vi "WaitMachine2OFF.vi"(10 "Station":string, 11 "SN":string="7510833") -> (0 "DupResult":string, 1 "Result":string, 2 "NGTag":string, 3 "Left/Right":string)   [LabVIEW 2020]
uses:
  <vilib>/Utility/config.llb/Read Key (String).vi
  <vilib>/Utility/config.llb/NI_LVConfig.lvlib
panel:
  out "Running":bool
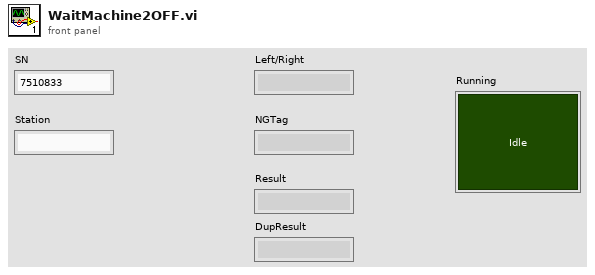
[diagram p1: front panel]
types:
  T1 = typedef "NI_LVConfig.lvlib/Config Data RefNum.ctl" = refnum<k1>
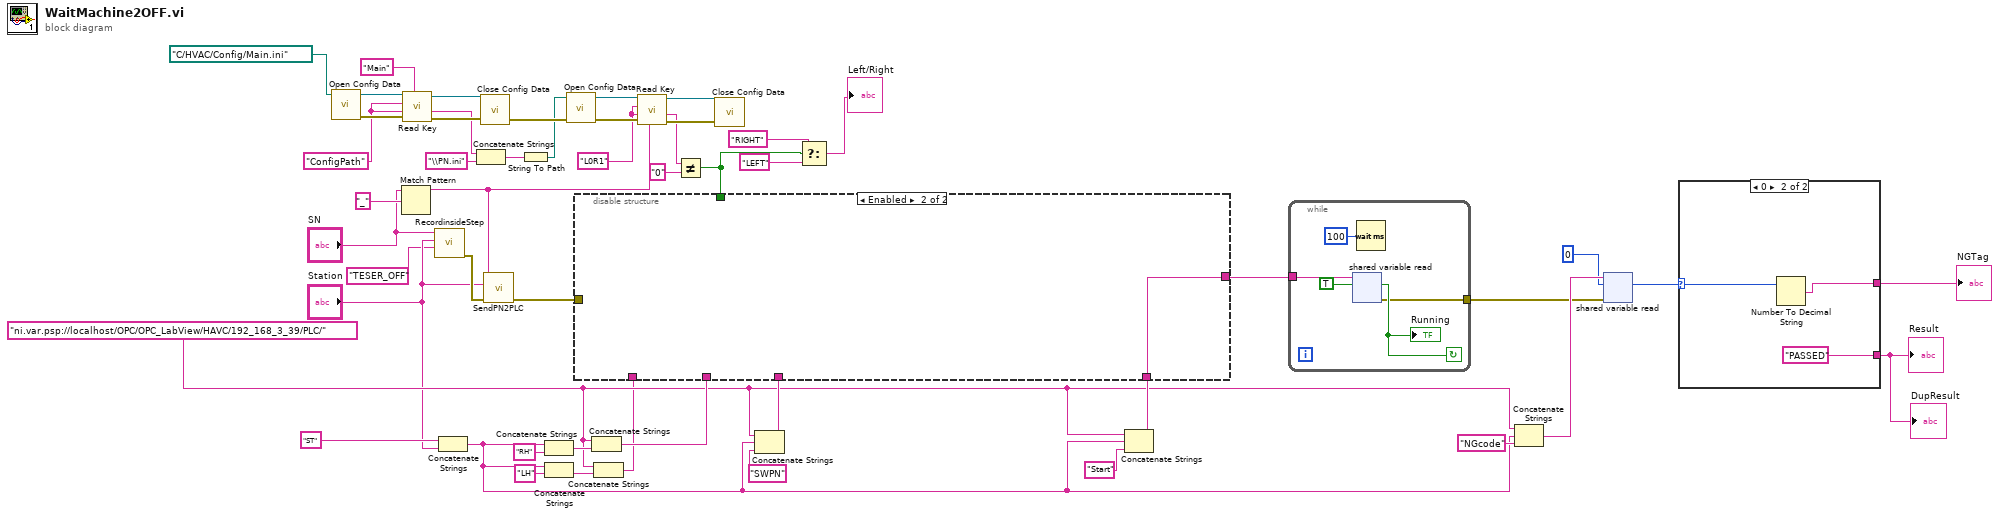
[diagram p0: block diagram]
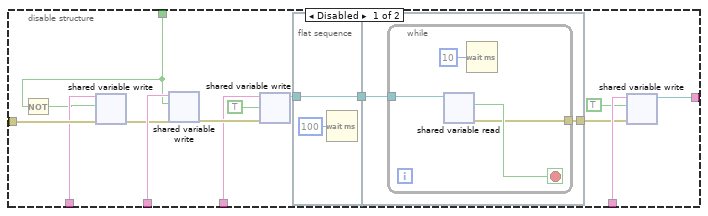
[diagram p2: hidden frame]
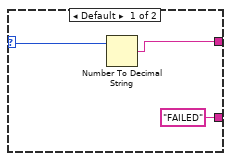
[diagram p3: hidden frame]
diagram:
  w31 = "L0R1"
  w45 = "ConfigPath" ("key")
  w10 = "ni.var.psp://localhost/OPC/OPC_LabView/HAVC/192_168_3_39/PLC/" ("string")
  n1 = call <vilib>:"Open Config Data.vi"("configuration file path"=path "C:/HVAC/Config/Main.ini") -> ("error out"=w50:errorcluster, "refnum"=w49:T1)  [unwired: 8 in, 1 out]
  n2 = Match Pattern(string="SN", regular expression="_") -> (before substring=w6:string)  [unwired: 1 in, 3 out]
  n3 = call-poly <vilib>:"Read Key.vi"("section"="Main", "error in (no error)"=w50, "default value"=w45, "key"=w45, "refnum"=w49) -> ("error out"=w47:errorcluster, "value"=w44:string, "refnum out"=w48:T1)  [unwired: 3 in, 1 out]
  n4 = call "RecordinsideStep.vi"("STEP"="TESER_OFF", "Station"="Station", "SN"="SN") -> ("error out"=w4:errorcluster)  [unwired: 8 in]
  n5 = Concatenate Strings("ST", "Station") -> (w13:string)
  n6 = Concatenate Strings(w44, "\\PN.ini" ("string")) -> (w37:string)
  n7 = call <vilib>:"Close Config Data.vi"("error in (no error)"=w47, "refnum"=w48) -> ("error out"=w38:errorcluster)  [unwired: 8 in, 1 out]
  n8 = call "SendPN2PLC.vi"("error in (no error)"=w4, "Station"="Station", "PN"=w6) -> ("error out"=w9:errorcluster)  [unwired: 7 in, 1 out]
  n9 = String To Path(string=w37) -> (path=w36:path)
  n10 = Concatenate Strings(w13, "RH" ("string")) -> (w33:string)
  n11 = Concatenate Strings(w13, "LH" ("string")) -> (w11:string)
  n12 = call <vilib>:"Open Config Data.vi"("error in (no error)"=w38, "configuration file path"=w36) -> ("error out"=w42:errorcluster, "refnum"=w41:T1)  [unwired: 7 in, 1 out]
  n13 = Concatenate Strings(w10, w33) -> (w32:string)
  n14 = Concatenate Strings(w10, w11) -> (w8:string)
  n15 = call-poly <vilib>:"Read Key.vi"("section"=w6, "error in (no error)"=w42, "default value"=w31, "key"=w31, "refnum"=w41) -> ("error out"=w39:errorcluster, "value"=w29:string, "refnum out"=w40:T1)  [unwired: 3 in, 1 out]
  n16 = Not Equal?(x=w29, y="0") -> (x != y?=w7:bool)
  n17 = call <vilib>:"Close Config Data.vi"("error in (no error)"=w39, "refnum"=w40) -> ()  [unwired: 8 in, 2 out]
  n18 = Concatenate Strings(w10, w13, "SWPN" ("string")) -> (w25:string)
  n19 = Select(t="RIGHT" ("y"), s=w7, f="LEFT" ("y")) -> (s? t:f=→"Left/Right":string)
  n20 = Concatenate Strings(w10, w13, "Start" ("string")) -> (w22:string)
  n21 = disable-structure shown="Enabled" {
    disable-tunnel: w32 -> [w65 _]
    disable-tunnel: w25 -> [w63 _]
    disable-tunnel: w22 -> [w60 w75]
    disable-tunnel: [w58 w75] -> w21
    disable-tunnel: w9 -> [w55 _]
    disable-tunnel: w8 -> [w54 _]
    disable-tunnel: w7 -> [w52 _]
    frame Disabled {
      n22 = Not(x=w52) -> (.not. x?=w53:bool)
      n23 = shared-variable-write(w54, w55, w53) -> (w56:errorcluster)  [unwired: 1 out]
      n24 = shared-variable-write(w65, w56, w52) -> (w64:errorcluster)  [unwired: 1 out]
      n25 = shared-variable-write(w63, w64, TRUE) -> (w61:refnum<k21>)  [unwired: 1 out]
      n26 = flat-sequence {
        tunnel: w61 -> [w68]
        tunnel: [w68] -> w66
        tunnel: [w69] -> w57
        tunnel: w66 -> [w70]
        frame #0 {
          n27 = Wait (ms)(milliseconds to wait=u32 100) -> ()  [unwired: 1 out]
        }
        frame #1 {
          n28 = while {
            tunnel: w70 -> [w74]
            tunnel: [w71] -> w69
            stop <- w72 stop-if-true
            n29 = shared-variable-read(w74) -> (w71:errorcluster, w72:bool)  [unwired: 1 in, 2 out]
            n30 = Wait (ms)(milliseconds to wait=u32 10) -> ()  [unwired: 1 out]
          }
        }
      }
      n31 = shared-variable-write(w60, w57, TRUE ("data in")) -> (w58:refnum<k21>)  [unwired: 1 out]
    }
    frame Enabled {
    }
  }
  n32 = while {
    tunnel: w21 -> [w79]
    tunnel: [w77] -> w18
    stop <- w78 continue-if-true
    n33 = shared-variable-read(w79, TRUE) -> (w77:errorcluster, w78:bool)  [unwired: 1 in, 2 out]
    "Running" <- w78
    n34 = Wait (ms)(milliseconds to wait=u32 100) -> ()  [unwired: 1 out]
  }
  n35 = Concatenate Strings(w10, w13, "NGcode" ("string")) -> (w19:string)
  n36 = shared-variable-read(w19, w18, 0) -> (w16:i32)  [unwired: 3 out]
  n37 = case shown="0" w16 {
    selector: w16 -> [w82 w85]
    tunnel: ["FAILED" "PASSED"] -> w14
    tunnel: [w81 w84] -> w15
    frame Default {
      n38 = Number To Decimal String(number=w82) -> (decimal integer string=w81:string)  [unwired: 1 in]
    }
    frame 0 {
      n39 = Number To Decimal String(number=w85) -> (decimal integer string=w84:string)  [unwired: 1 in]
    }
  }
  "NGTag" <- w15
  "Result" <- w14
  "DupResult" <- w14
